vi "Swerve Tracker 2020.vi"(11 "Calibration Constant":i32=12000000) -> ()   [LabVIEW 2018]
uses:
  Robot Global Data.vi
  <vilib>/Rock Robotics/WPI/ThirdParty/Phoenix-LabVIEW/Motor Controller/Get/CTRE_Phoenix_MotorController_GetSelectedSensorData.vi
  <vilib>/Rock Robotics/Network Tables/NT Write Numeric Array.vi
  <vilib>/ptbypt/NI_PtbyPt.lvlib
panel:
  out "Drive Encoders":dbl[](array[numeric])
  out "Loop 2":u32=31
  # "SWERVE DRIVE\nVersion 7.1\nCory Lynch\nChris Garuti\nGavin Popkin\nKaitlyn Sandor\nEthan Silver\nApple Pi Robotics\nTeam 2067"
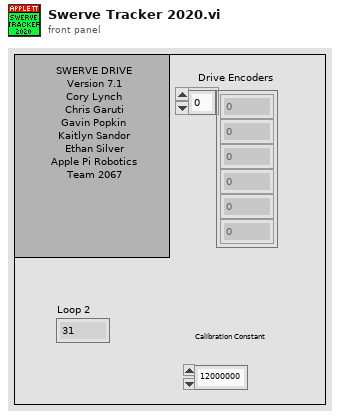
[diagram p1: front panel]
types:
  T1 = enum16{"Sparkmax Brushless", "Talon SRX Brushed"}
  T2 = typedef "WPI_MotorControlDeviceRef.ctl" = cluster{"DeviceStatus":errorcluster, "Type":T3, "PWM":cluster{"PWM Channel":T4, "DeadBand":T5}, "CAN":cluster{"Device Number":u8, "SetOutput VI Ref":variant, "GetOutput VI Ref":variant, "Enable VI Ref":variant, "Disable VI Ref":variant, "Data":variant}, "Invert":bool, "DIO PWM":cluster{"PWM \"Enable\" Channel":T4, "DIOChannel":T6, "PWM Rate":dbl}}
  T3 = typedef "WPI_MotorControlType.ctl" = enum16{"PWM", "CAN", "DIO PWM"}
  T4 = typedef "FPGA_DIOPWMChannel.ctl" = enum8{"PWM 0", "PWM 1", "PWM 2", "PWM 3", "PWM 4", "PWM 5", "PWM 6", "PWM 7", "PWM 8", "PWM 9", "PWM MXP 0", "PWM MXP 1", "PWM MXP 2", "PWM MXP 3", "PWM MXP 4", "PWM MXP 5", "PWM MXP 6", "PWM MXP 7", "PWM MXP 8", "PWM MXP 9", "Invalid"}
  T5 = typedef "WPI_PWMDeadband.ctl" = cluster{"Name":string, "maxPositivePwm":i32, "minPositivePwm":i32, "centerPwm":i32, "maxNegativePwm":i32, "minNegativePwm":i32, "angularRange":u16}
  T6 = typedef "FPGA_DIOChannel.ctl" = enum8{"DIO 0", "DIO 1", "DIO 2", "DIO 3", "DIO 4", "DIO 5", "DIO 6", "DIO 7", "DIO 8", "DIO 9", "DIO MXP 0", "DIO MXP 1", "DIO MXP 2", "DIO MXP 3", "DIO MXP 4", "DIO MXP 5", "DIO MXP 6", "DIO MXP 7", "DIO MXP 8", "DIO MXP 9", "DIO MXP 10", "DIO MXP 11", "DIO MXP 12", "DIO MXP 13", "DIO MXP 14", "DIO MXP 15", "SPI Port CS1", "SPI Port CS2", "SPI Port CS3", "SPI Port MISO", "SPI Port MOSI", "Invalid"}
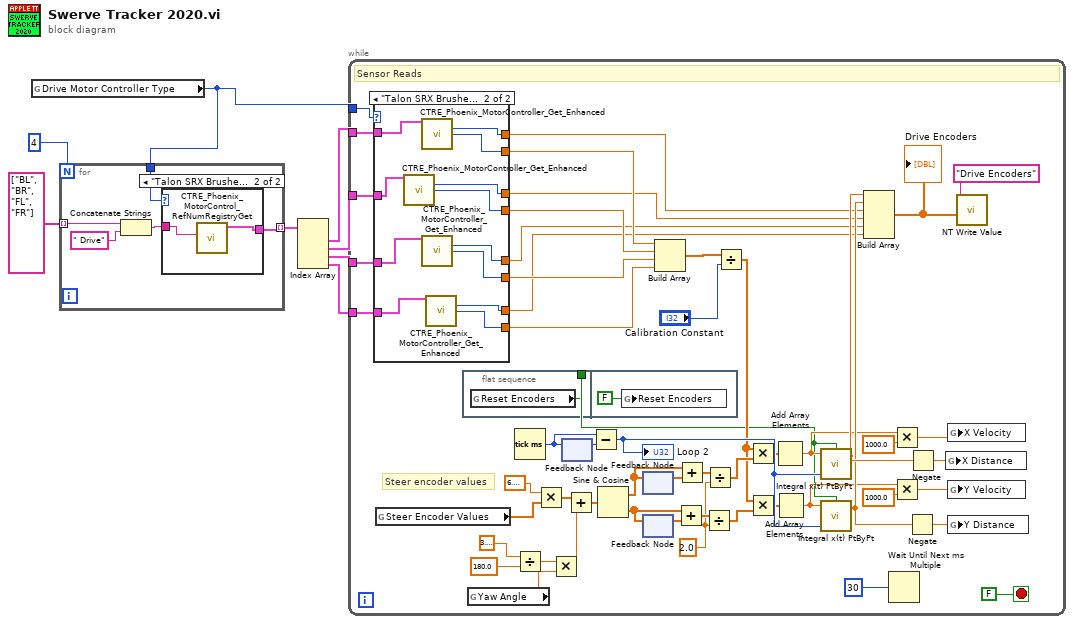
[diagram p0: block diagram]
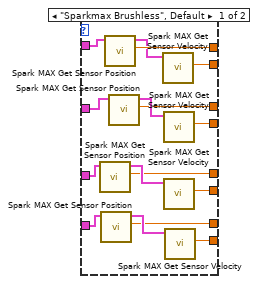
[diagram p2: hidden frame]
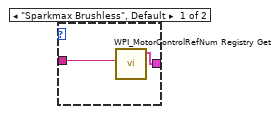
[diagram p3: hidden frame]
diagram:
  n1 = global read "Robot Global Data.vi" "Drive Motor Controller Type"() -> (w1:T1)
  n2 = for {
    N: 4 -> [_]
    tunnel: string[] ["BL", "BR", "FL", "FR"] -> [w13] mode=indexing
    tunnel: [w11] -> w2 mode=indexing
    tunnel: w1 -> [w9]
    n3 = Concatenate Strings(w13, " Drive") -> (w10:string)
    n4 = case shown="\"Talon SRX Brushed\"" w9 {
      tunnel: [w15 w16] -> w11
      tunnel: w10 -> [w14 w17]
      frame "Sparkmax Brushless", Default {
        n5 = call <vilib>:"WPI_MotorControlRefNum Registry Get.vi"("refnum name"=w14) -> ("MotorControlDevRef"=w15:T2)  [unwired: 9 in, 1 out]
      }
      frame "Talon SRX Brushed" {
        n6 = call <vilib>:"CTRE_Phoenix_MotorControl_RefNumRegistryGet.vi"("refnum name"=w17) -> ("PhoenixMotorControlDevRef"=w16:T2)  [unwired: 9 in, 1 out]
      }
    }
  }
  n7 = Index Array(array=w2) -> (element #1=w6:T2, element #2=w5:T2, element #3=w4:T2, element #4=w3:T2)  [unwired: 4 in]
  n8 = while {
    tunnel: w6 -> [w31]
    tunnel: w5 -> [w29]
    tunnel: w4 -> [w26]
    tunnel: w3 -> [w24]
    tunnel: w1 -> [w18]
    stop <- FALSE stop-if-true
    w42 = 2.0
    # "Steer encoder values"
    # "Sensor Reads"
    n9 = case shown="\"Talon SRX Brushed\"" w18 {
      tunnel: [w87 w98] -> w32
      tunnel: w31 -> [w86 w99]
      tunnel: [w85 w97] -> w30
      tunnel: w29 -> [w82 w96]
      tunnel: [w81 w95] -> w28
      tunnel: [w80 w94] -> w27
      tunnel: w26 -> [w78 w93]
      tunnel: [w77 w92] -> w25
      tunnel: w24 -> [w75 w90]
      tunnel: [w74 w91] -> w23
      tunnel: [w73 w89] -> w22
      tunnel: [w72 w88] -> w21
      frame "Sparkmax Brushless", Default {
        n10 = call <vilib>:"Spark MAX Get Sensor Position.vi"("MotorControlDevRef in"=w78) -> ("Sensor Position"=w77:dbl, "MotorControlDevRef out"=w79:T2)  [unwired: 7 in, 2 out]
        n11 = call <vilib>:"Spark MAX Get Sensor Position.vi"("MotorControlDevRef in"=w75) -> ("Sensor Position"=w73:dbl, "MotorControlDevRef out"=w76:T2)  [unwired: 7 in, 2 out]
        n12 = call <vilib>:"Spark MAX Get Sensor Position.vi"("MotorControlDevRef in"=w86) -> ("Sensor Position"=w87:dbl, "MotorControlDevRef out"=w84:T2)  [unwired: 7 in, 2 out]
        n13 = call <vilib>:"Spark MAX Get Sensor Position.vi"("MotorControlDevRef in"=w82) -> ("Sensor Position"=w81:dbl, "MotorControlDevRef out"=w83:T2)  [unwired: 7 in, 2 out]
        n14 = call <vilib>:"Spark MAX Get Sensor Velocity.vi"("MotorControlDevRef in"=w84) -> ("Sensor Velocity"=w85:dbl)  [unwired: 7 in, 3 out]
        n15 = call <vilib>:"Spark MAX Get Sensor Velocity.vi"("MotorControlDevRef in"=w83) -> ("Sensor Velocity"=w80:dbl)  [unwired: 7 in, 3 out]
        n16 = call <vilib>:"Spark MAX Get Sensor Velocity.vi"("MotorControlDevRef in"=w79) -> ("Sensor Velocity"=w74:dbl)  [unwired: 7 in, 3 out]
        n17 = call <vilib>:"Spark MAX Get Sensor Velocity.vi"("MotorControlDevRef in"=w76) -> ("Sensor Velocity"=w72:dbl)  [unwired: 7 in, 3 out]
      }
      frame "Talon SRX Brushed" {
        n18 = call-poly <vilib>:"CTRE_Phoenix_MotorController_Get_Enhanced.vi"("PhoenixMotorControlDevRef"=w96) -> ("Position (Raw Sensor Units)"=w95:i32, "Velocity (Raw Sensor Units per 100 ms)"=w94:i32)  [unwired: 11 in, 2 out]
        n19 = call-poly <vilib>:"CTRE_Phoenix_MotorController_Get_Enhanced.vi"("PhoenixMotorControlDevRef"=w99) -> ("Position (Raw Sensor Units)"=w98:i32, "Velocity (Raw Sensor Units per 100 ms)"=w97:i32)  [unwired: 11 in, 2 out]
        n20 = call-poly <vilib>:"CTRE_Phoenix_MotorController_Get_Enhanced.vi"("PhoenixMotorControlDevRef"=w93) -> ("Position (Raw Sensor Units)"=w92:i32, "Velocity (Raw Sensor Units per 100 ms)"=w91:i32)  [unwired: 11 in, 2 out]
        n21 = call-poly <vilib>:"CTRE_Phoenix_MotorController_Get_Enhanced.vi"("PhoenixMotorControlDevRef"=w90) -> ("Position (Raw Sensor Units)"=w89:i32, "Velocity (Raw Sensor Units per 100 ms)"=w88:i32)  [unwired: 11 in, 2 out]
      }
    }
    n22 = global read "Robot Global Data.vi" "Steer Encoder Values"() -> (w19:dbl[])
    n23 = flat-sequence {
      tunnel: [w100] -> w35
      frame #0 {
        n24 = global read "Robot Global Data.vi" "Reset Encoders"() -> (w100:bool)
      }
      frame #1 {
        n25 = global write "Robot Global Data.vi" "Reset Encoders"(FALSE ("Reset Encoders")) -> ()
      }
    }
    n26 = global read "Robot Global Data.vi" "Yaw Angle"() -> (w20:dbl)
    n27 = Tick Count (ms)() -> (millisecond timer value=w69:u32)
    n28 = Divide(x=3.141592653589793, y=180.0) -> (x/y=w62:dbl)
    n29 = Multiply(x=6.283185307179586, y=w19) -> (x*y=w65:dbl[])
    n30 = Multiply(x=w62, y=w20) -> (x*y=w61:dbl)
    n31 = feedback #1() -> (w68:u32)  [unwired: 1 in]
    n32 = feedback-in #1(w69) -> ()
    n33 = Add(x=w65, y=w61) -> (x+y=w66:dbl[])
    n34 = Subtract(x=w69, y=w68) -> (x-y=w58:u32)
    "Loop 2" <- w58
    n35 = Sine & Cosine(0:w66) -> (1:w48:dbl[], 2:w43:dbl[])
    n36 = feedback #2() -> (w49:dbl[])  [unwired: 1 in]
    n37 = feedback-in #2(w48) -> ()
    n38 = feedback #3() -> (w44:dbl[])  [unwired: 1 in]
    n39 = feedback-in #3(w43) -> ()
    n40 = Build Array(w30, w27, w23, w21) -> (w39:dbl[])
    n41 = Add(x=w43, y=w44) -> (x+y=w45:dbl[])
    n42 = Add(x=w48, y=w49) -> (x+y=w46:dbl[])
    n43 = Divide(x=w45, y=w42) -> (x/y=w41:dbl[])
    n44 = Divide(x=w46, y=w42) -> (x/y=w47:dbl[])
    n45 = Divide(x=w39, y="Calibration Constant") -> (x/y=w36:dbl[])
    n46 = Multiply(x=w36, y=w47) -> (x*y=w57:dbl[])
    n47 = Multiply(x=w36, y=w41) -> (x*y=w56:dbl[])
    n48 = Add Array Elements(numeric array=w57) -> (sum=w53:dbl)
    n49 = Add Array Elements(numeric array=w56) -> (sum=w52:dbl)
    n50 = call <vilib>:"Integral x(t) PtByPt.vi"("initialize"=w35, "dt"=w58, "x"=w53) -> ("integral x(t)"=w60:dbl)  [unwired: 1 in, 1 out]
    n51 = call <vilib>:"Integral x(t) PtByPt.vi"("initialize"=w35, "dt"=w58, "x"=w52) -> ("integral x(t)"=w59:dbl)  [unwired: 1 in, 1 out]
    n52 = Build Array(w60, w59, w32, w28, w25, w22) -> (w38:dbl[])
    "Drive Encoders" <- w38
    n53 = Wait Until Next ms Multiple(millisecond multiple=u32 30) -> ()  [unwired: 1 out]
    n54 = Multiply(x=w53, y=1000.0) -> (x*y=w51:dbl)
    n55 = Multiply(x=w52, y=1000.0) -> (x*y=w50:dbl)
    n56 = Negate(x=w59) -> (-x=w34:dbl)
    n57 = Negate(x=w60) -> (-x=w33:dbl)
    n58 = global write "Robot Global Data.vi" "X Distance"(w33) -> ()
    n59 = global write "Robot Global Data.vi" "X Velocity"(w51) -> ()
    n60 = global write "Robot Global Data.vi" "Y Velocity"(w50) -> ()
    n61 = global write "Robot Global Data.vi" "Y Distance"(w34) -> ()
    n62 = call-poly <vilib>:"NT Write Value.vi"("Numeric Array"=w38, "Name"="Drive Encoders") -> ()  [unwired: 9 in, 1 out]
  }
